vi "computer max min & gains.vi"(10 "Sensor":T2={"manner"=enum."线性", "data"=[[1.0, 0.0], [1.0, 2.0], [2.0, 4.0], [3.0, 6.0], [5.0, 10.0], [6.0, 12.0], [12.0, 24.0], [13.0, 26.0]], "slop"=10.0, "intercept"=-10.0, "sensorID"="Vi", "signal type"="加速度", "unit"="g"}) -> (0 "gains":string, 1 "b value":string, 2 "k value":string)   [LabVIEW 2011]
uses:
  gain.ctl
  <vilib>/Analysis/NI_AALPro.lvlib
panel:
  in  "Gain":T1
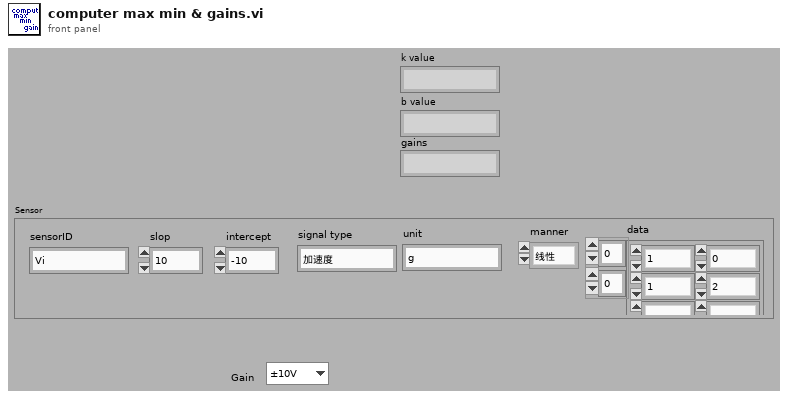
[diagram p1: front panel]
types:
  T1 = typedef "gain.ctl" = enum16{"±10V", "±5V", "±2.5V", "±1V", "±500mV", "±100mV", "10V", "5V", "2.5V", "1V", "500mV", "100mV"}
  T2 = cluster{"manner":enum16{"线性", "查表"}, "data":dbl[][], "slop":dbl, "intercept":dbl, "sensorID":string, "signal type":string, "unit":string}
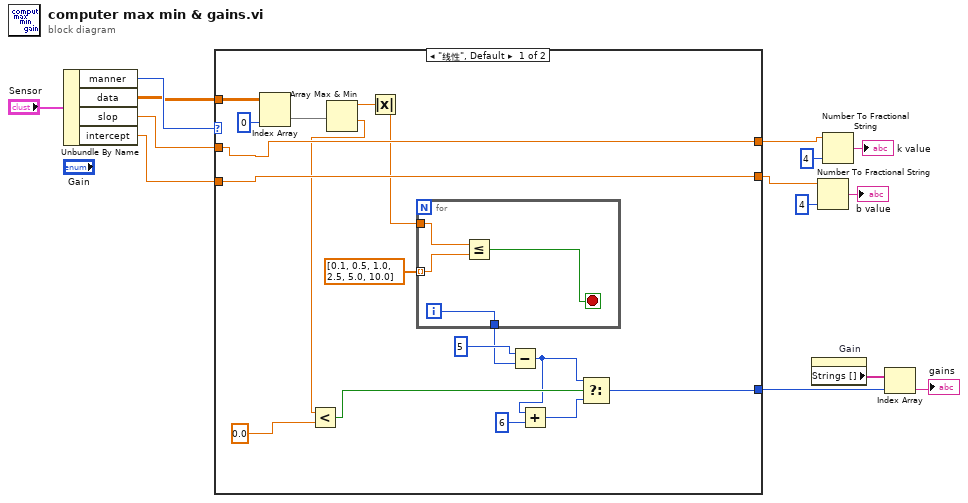
[diagram p0: block diagram]
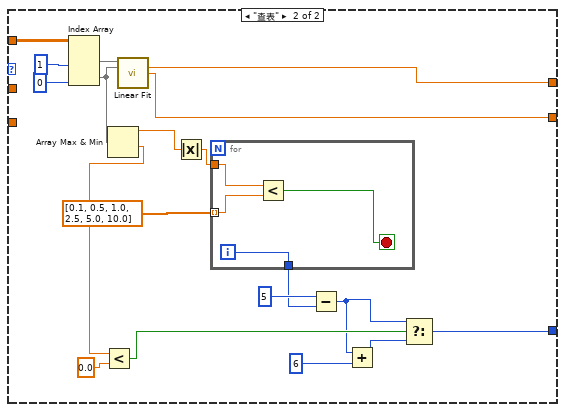
[diagram p2: hidden frame]
diagram:
  n1 = Unbundle By Name("Sensor") -> ("manner"=w13:enum16{"线性", "查表"}, "data"=w12:dbl[][], "slop"=w11:dbl, "intercept"=w10:dbl)
  n2 = case shown="\"线性\", Default" w13 {
    tunnel: w12 -> [w20 w40]
    tunnel: w11 -> [w22 _]
    tunnel: w10 -> [w21 _]
    tunnel: [w22 w44] -> w7
    tunnel: [w21 w43] -> w6
    tunnel: [w23 w46] -> w9
    frame "线性", Default {
      n3 = Index Array(array=w20, index (col)=0 ("disabled index (col)")) -> (element=w18:dbl[])  [unwired: 1 in]
      n4 = Array Max & Min(array=w18) -> (max value=w17:dbl, min value=w15:dbl)  [unwired: 2 out]
      n5 = Less?(x=w15, y=0.0) -> (x < y?=w27:bool)
      n6 = Absolute Value(x=w17) -> (abs(x)=w16:dbl)
      n7 = for {
        tunnel: w16 -> [w35]
        tunnel: dbl[] [0.1, 0.5, 1.0, 2.5, 5.0, 10.0] -> [w34] mode=indexing
        tunnel: [w32] -> w28
        i -> [w32]
        stop <- w33 stop-if-true
        n8 = Less Or Equal?(x=w35, y=w34) -> (x <= y?=w33:bool)
      }
      n9 = Subtract(x=5 ("y"), y=w28) -> (x-y=w25:i32)
      n10 = Add(x=w25, y=6) -> (x+y=w26:i32)
      n11 = Select(t=w25, s=w27, f=w26) -> (s? t:f=w23:i32)
    }
    frame "查表" {
      n12 = Index Array(array=w40, index (col) #1=1 ("disabled index (col)"), index (col) #2=0 ("index (col)")) -> (element #1=w45:dbl[], element #2=w39:dbl[])  [unwired: 2 in]
      n13 = Array Max & Min(array=w39) -> (max value=w38:dbl, min value=w36:dbl)  [unwired: 2 out]
      n14 = Less?(x=w36, y=0.0) -> (x < y?=w50:bool)
      n15 = call <vilib>:"Linear Fit.vi"("Y"=w45, "X"=w39) -> ("slope"=w44:dbl, "intercept"=w43:dbl)  [unwired: 4 in, 8 out]
      n16 = Absolute Value(x=w38) -> (abs(x)=w37:dbl)
      n17 = for {
        tunnel: w37 -> [w58]
        tunnel: dbl[] [0.1, 0.5, 1.0, 2.5, 5.0, 10.0] -> [w57] mode=indexing
        tunnel: [w55] -> w51
        i -> [w55]
        stop <- w56 stop-if-true
        n18 = Less?(x=w58, y=w57) -> (x < y?=w56:bool)
      }
      n19 = Subtract(x=5 ("y"), y=w51) -> (x-y=w48:i32)
      n20 = Add(x=w48, y=6) -> (x+y=w49:i32)
      n21 = Select(t=w48, s=w50, f=w49) -> (s? t:f=w46:i32)
    }
  }
  n22 = property on="Gain" class="Enum (strict)"() -> ("Strings []"=w8:string[])  [unwired: 2 in, 2 out]
  n23 = Number To Fractional String(number=w6, precision (6)=i16 4) -> (F-format string=→"b value":string)  [unwired: 2 out]
  n24 = Number To Fractional String(number=w7, precision (6)=i16 4) -> (F-format string=→"k value":string)  [unwired: 2 out]
  n25 = Index Array(array=w8, index=w9) -> (element=→"gains":string)
